vi "Test_serial.vi"(6 "VISA resource name":refnum<visa-resource-name>, 7 "Passed so far?":bool, 8 "error in (no error)":errorcluster, 11 "Slot":T1) -> (0 "error out":errorcluster, 2 "read buffer":string, 4 "VISA resource name out":refnum<visa-resource-name>, 5 "Passed?":bool)   [LabVIEW 2024]
uses:
  AP slots to test.ctl
  <vilib>/Utility/error.llb/Trim Whitespace One-Sided.vi
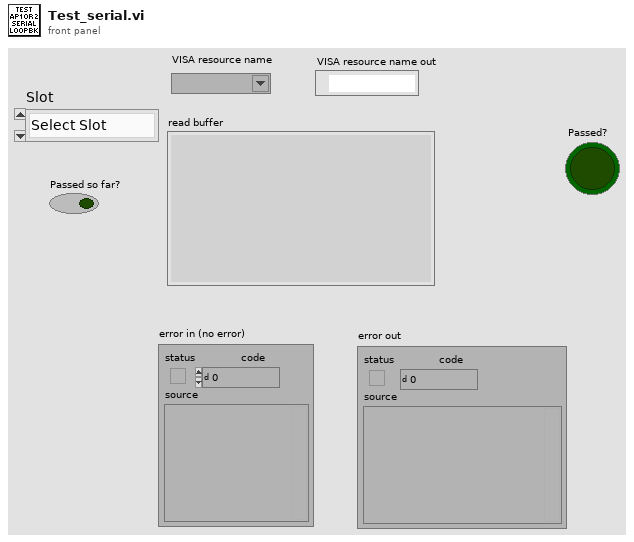
[diagram p1: front panel]
types:
  T1 = typedef "AP slots to test.ctl" = enum16{"Select Slot", "AP1", "AP2", "AP1 and AP2"}
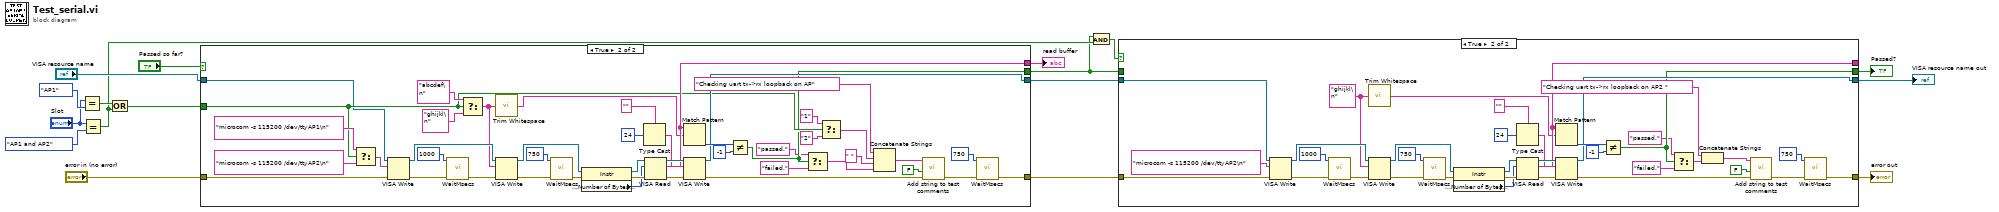
[diagram p0: block diagram]
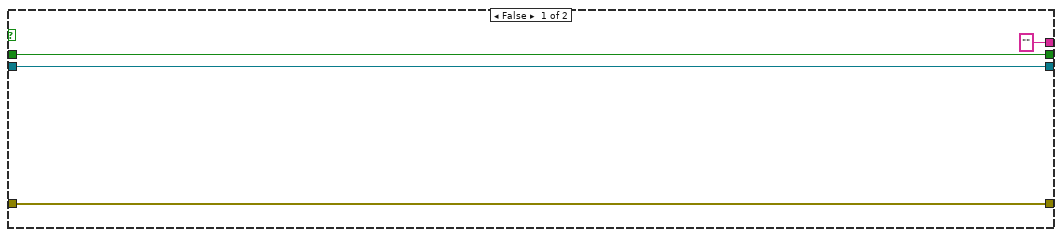
[diagram p2: hidden frame]
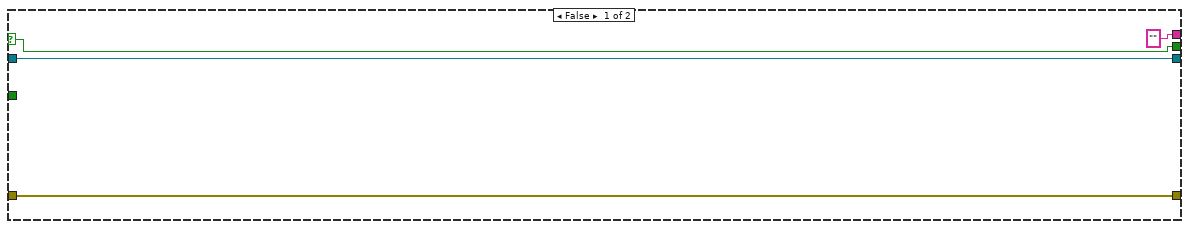
[diagram p3: hidden frame]
diagram:
  n1 = Equal?(x="Slot", y=AP_slots_to_test."AP1") -> (x = y?=w12:bool)
  n2 = Equal?(x="Slot", y=AP_slots_to_test."AP1 and AP2") -> (x = y?=w3:bool)
  n3 = Or(x=w12, y=w3) -> (x .or. y?=w11:bool)
  n4 = case shown="True" "Passed so far?" {
    selector: "Passed so far?" -> [w19 _]
    tunnel: "error in (no error)" -> [w21 w26]
    tunnel: [w21 w22] -> w6
    tunnel: ["" ("read buffer") w50] -> w16
    tunnel: [w19 w31] -> w1
    tunnel: w11 -> [_ w36]
    tunnel: "VISA resource name" -> [w20 w25]
    tunnel: [w20 w40] -> w7
    frame False {
    }
    frame True {
      n5 = Select(t="microcom -s 115200 /dev/ttyAP1\n", s=w36, f="microcom -s 115200 /dev/ttyAP2\n") -> (s? t:f=w45:string)
      n6 = VISA Write(VISA resource name=w25, write buffer=w45, error in (no error)=w26) -> (VISA resource name out=w52:refnum<visa-resource-name>, error out=w53:errorcluster)  [unwired: 1 out]
      n7 = call "WaitMsecs.vi"("error in (no error)"=w53, "Wait Msecs"=u32 1000) -> ("error out"=w51:errorcluster)  [unwired: 9 in]
      n8 = Select(t="abcdef\n" ("write buffer"), s=w36, f="ghijkl\n" ("write buffer")) -> (s? t:f=w42:string)
      n9 = call <vilib>:"Trim Whitespace.vi"("string"=w42) -> ("trimmed string"=w41:string)  [unwired: 1 in]
      n10 = VISA Write(VISA resource name=w52, write buffer=w42, error in (no error)=w51) -> (VISA resource name out=w60:refnum<visa-resource-name>, error out=w61:errorcluster)  [unwired: 1 out]
      n11 = call "WaitMsecs.vi"("error in (no error)"=w61, "Wait Msecs"=u32 750) -> ("error out"=w65:errorcluster)  [unwired: 9 in]
      n12 = property class="Instr"(reference=w60, error in=w65) -> (reference out=w64:refnum<visa-resource-name>, error out=w63:errorcluster, "Serial Settings:Number of Bytes at Serial Port"=w62:u32)
      n13 = Type Cast(type="" ("write buffer"), x=24) -> (*(type *) &x=w55:string)
      n14 = VISA Read(VISA resource name=w64, byte count=w62, error in (no error)=w63) -> (VISA resource name out=w58:refnum<visa-resource-name>, read buffer=w50:string, error out=w59:errorcluster)  [unwired: 1 out]
      n15 = Match Pattern(string=w50, regular expression=w41) -> (offset past match=w49:i32)  [unwired: 1 in, 3 out]
      n16 = VISA Write(VISA resource name=w58, write buffer=w55, error in (no error)=w59) -> (VISA resource name out=w40:refnum<visa-resource-name>, error out=w38:errorcluster)  [unwired: 1 out]
      n17 = Not Equal?(x=w49, y=-1) -> (x != y?=w31:bool)
      n18 = Select(t="passed.", s=w31, f="failed.") -> (s? t:f=w28:string)
      n19 = Select(t="1", s=w36, f="2") -> (s? t:f=w33:string)
      n20 = Concatenate Strings("Checking uart tx->rx loopback on AP" ("string"), w33, " " ("string"), w28) -> (w27:string)
      n21 = call "Add string to test comments.vi"("error in (no error)"=w38, "New Section (y)?"=FALSE, "Comments"=w27) -> ("error out"=w23:errorcluster)  [unwired: 7 in, 1 out]
      n22 = call "WaitMsecs.vi"("error in (no error)"=w23, "Wait Msecs"=u32 750) -> ("error out"=w22:errorcluster)  [unwired: 9 in]
    }
  }
  "read buffer" <- w16
  n23 = And(x=w1, y=w3) -> (x .and. y?=w2:bool)
  n24 = case shown="True" w2 {
    tunnel: w6 -> [w70 w77]
    tunnel: [w70 w73] -> w8
    tunnel: ["" ("read buffer") w90] -> _
    tunnel: [w67 w82] -> w4
    tunnel: w7 -> [w69 w76]
    tunnel: [w69 w86] -> w5
    tunnel: w1 -> [w67 _]
    frame False {
    }
    frame True {
      w71 = "ghijkl\n" ("write buffer")
      n25 = VISA Write(VISA resource name=w76, write buffer="microcom -s 115200 /dev/ttyAP2\n", error in (no error)=w77) -> (VISA resource name out=w92:refnum<visa-resource-name>, error out=w93:errorcluster)  [unwired: 1 out]
      n26 = call "WaitMsecs.vi"("error in (no error)"=w93, "Wait Msecs"=u32 1000) -> ("error out"=w91:errorcluster)  [unwired: 9 in]
      n27 = call <vilib>:"Trim Whitespace.vi"("string"=w71) -> ("trimmed string"=w87:string)  [unwired: 1 in]
      n28 = VISA Write(VISA resource name=w92, write buffer=w71, error in (no error)=w91) -> (VISA resource name out=w100:refnum<visa-resource-name>, error out=w101:errorcluster)  [unwired: 1 out]
      n29 = call "WaitMsecs.vi"("error in (no error)"=w101, "Wait Msecs"=u32 750) -> ("error out"=w105:errorcluster)  [unwired: 9 in]
      n30 = property class="Instr"(reference=w100, error in=w105) -> (reference out=w104:refnum<visa-resource-name>, error out=w103:errorcluster, "Serial Settings:Number of Bytes at Serial Port"=w102:u32)
      n31 = Type Cast(type="" ("write buffer"), x=24) -> (*(type *) &x=w95:string)
      n32 = VISA Read(VISA resource name=w104, byte count=w102, error in (no error)=w103) -> (VISA resource name out=w98:refnum<visa-resource-name>, read buffer=w90:string, error out=w99:errorcluster)  [unwired: 1 out]
      n33 = Match Pattern(string=w90, regular expression=w87) -> (offset past match=w89:i32)  [unwired: 1 in, 3 out]
      n34 = VISA Write(VISA resource name=w98, write buffer=w95, error in (no error)=w99) -> (VISA resource name out=w86:refnum<visa-resource-name>, error out=w84:errorcluster)  [unwired: 1 out]
      n35 = Not Equal?(x=w89, y=-1) -> (x != y?=w82:bool)
      n36 = Select(t="passed.", s=w82, f="failed.") -> (s? t:f=w79:string)
      n37 = Concatenate Strings("Checking uart tx->rx loopback on AP2 " ("string"), w79) -> (w78:string)
      n38 = call "Add string to test comments.vi"("error in (no error)"=w84, "New Section (y)?"=FALSE, "Comments"=w78) -> ("error out"=w74:errorcluster)  [unwired: 7 in, 1 out]
      n39 = call "WaitMsecs.vi"("error in (no error)"=w74, "Wait Msecs"=u32 750) -> ("error out"=w73:errorcluster)  [unwired: 9 in]
    }
  }
  "error out" <- w8
  "Passed?" <- w4
  "VISA resource name out" <- w5
